vi "Swerve Controller.vi"(8 "error in":errorcluster) -> ()   [LabVIEW 2023]
doc: "This VI executes continuously carrying out the current operation and responding to updates or new operations. It will often contain the timing or control code that is difficult to place directly in TeleOp. This VI generally opens all sensors and motors and isolates the rest of the robot code from knowing how the operations are carried out."
uses:
  <vilib>/Rock Robotics/WPI/Framework/Completion Status.ctl
  Swerve Setpoints2.ctl
  Swerve Operations.ctl
  Framework/Robot Global Data.vi
  <vilib>/addons/control/pid/pid.llb/PID (DBL).vi
  <vilib>/addons/control/pid/NI_PID_pid.lvlib
  <vilib>/Rock Robotics/Network Tables/NT Write Boolean.vi
panel:
  out "error out":errorcluster
  out "x-y":u32
  in  "Tape":T1={"proportional gain (Kc)"=1.0, "integral time (Ti, min)"=0.01, "derivative time (Td, min)"=0.0} {"derivative time (Td, min)" format="%.3f"; "integral time (Ti, min)" format="%.3f"; "proportional gain (Kc)" format="%.3f"}
  in  "AprilTag":T1={"proportional gain (Kc)"=1.0, "integral time (Ti, min)"=0.01, "derivative time (Td, min)"=0.0} {"derivative time (Td, min)" format="%.3f"; "integral time (Ti, min)" format="%.3f"; "proportional gain (Kc)" format="%.3f"}
  in  "Look At Cube":T1={"proportional gain (Kc)"=0.001, "integral time (Ti, min)"=0.0, "derivative time (Td, min)"=0.0}
  in  "Look At Cone":T1={"proportional gain (Kc)"=0.004, "integral time (Ti, min)"=0.0, "derivative time (Td, min)"=0.01}
  in  "Balance":T1={"proportional gain (Kc)"=0.011, "integral time (Ti, min)"=0.0, "derivative time (Td, min)"=0.0} {"derivative time (Td, min)" format="%.3f"; "integral time (Ti, min)" format="%.3f"; "proportional gain (Kc)" format="%.3f"}
  in  "Drive to Angle(Distance)":T1={"proportional gain (Kc)"=0.9, "integral time (Ti, min)"=0.0, "derivative time (Td, min)"=0.0} {"derivative time (Td, min)" format="%.3f"; "integral time (Ti, min)" format="%.3f"; "proportional gain (Kc)" format="%.3f"}
  in  "Drive to Angle(Distance)":T1={"proportional gain (Kc)"=0.022, "integral time (Ti, min)"=0.0, "derivative time (Td, min)"=0.0} {"derivative time (Td, min)" format="%.3f"; "integral time (Ti, min)" format="%.3f"; "proportional gain (Kc)" format="%.3f"}
  out "Gyro":dbl
  in  "Drive to angle(Time)":T1={"proportional gain (Kc)"=0.019999999999999574, "integral time (Ti, min)"=0.0, "derivative time (Td, min)"=0.0} {"derivative time (Td, min)" format="%.3f"; "integral time (Ti, min)" format="%.3f"; "proportional gain (Kc)" format="%.3f"}
  in  "Turn to Angle":T1={"proportional gain (Kc)"=0.019999999999999574, "integral time (Ti, min)"=0.0, "derivative time (Td, min)"=0.0} {"derivative time (Td, min)" format="%.3f"; "integral time (Ti, min)" format="%.3f"; "proportional gain (Kc)" format="%.3f"}
  in  "Interactive Values":T2
  out "Current\nCmd":string="Started at  16:27:40.452\nDefault: Reserve,  S 0.0, D 0.000000"
  in  "Buttons":cluster{"Execute Cmd":bool, "Abort Cmd":bool}
  out "Command Timing":cluster{"Start Time (ms)":u32, "Iterations":i32}={"Start Time (ms)"=1585114, "Iterations"=-1}
  out "Status":T4=enum."Aborted"
  # "Tip: It may be helpful to observe inputs and sensor values.\nYou may also want to display tuning or debugging controls."
  # "Interactive Command: You may fill in the settings for a command\nand schedule it with the Execute button. You can observe and abort\nany command while fine tuning the code for the controller."
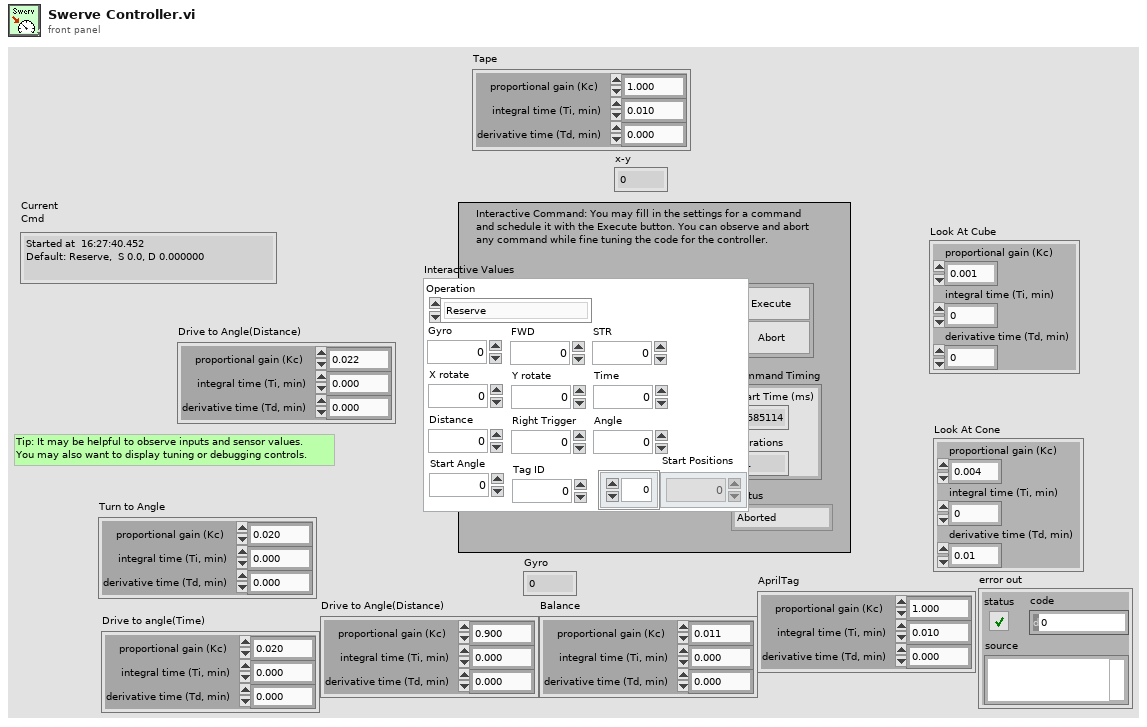
[diagram p1: front panel]
types:
  T1 = cluster{"proportional gain (Kc)":dbl, "integral time (Ti, min)":dbl, "derivative time (Td, min)":dbl}
  T2 = typedef "Swerve Setpoints2.ctl" = cluster{"Operation":T3, "Gyro":dbl, "FWD":dbl, "STR":dbl, "X rotate":dbl, "Y rotate":dbl, "Time":dbl, "Distance":dbl, "Right Trigger":dbl, "Angle":dbl, "Start Angle":dbl, "Tag ID":dbl, "Start Positions":dbl[]}
  T3 = typedef "Swerve Operations.ctl" = enum16{"Reserve", "Read Current", "Immediate", "Stop", "Balance", "Direct  Joystick Drive", "Joystick Drive", "Drive for Distance", "Drive for Time", "Turn to Angle", "Drive to Angle(Time)", "Drive to Angle(Distance)", "Look At Cone", "Look At Cube", "Move To Tape", "Move To Tag"}
  T4 = typedef "Completion Status.ctl" = enum16{"Successful", "Aborted", "Incomplete"}
  T5 = typedef "Command Status Info.ctl" = cluster{"Name":string, "Status":T4, "notifier out":T6}
  T6 = typedef "Completion Notifier.ctl" = refnum<notifier>
  T7 = cluster{"Current Command":T2, "Command Timing":cluster{"Start Time (ms)":u32, "Iterations":i32}, "Command Arguments":cluster{"Command Info":T5, "Description":string, "Default Command":T2, "queue out":refnum<queue>, "Subsystem Name":string}}
  T8 = enum16{"AprilTag", "Reflective Tape", "Custom", "Cube", "Cone"}
  T9 = typedef "ADIS16470 Device Reference.ctl" = cluster{"DevStatus":errorcluster, "Hardware Config":T10, "Calibration Complete":refnum<notifier>, "Status Reference":refnum<data-value>, "Data Reference":refnum<data-value>, "Sychronous Process VI":T14, "Cmd FIFO":refnum<k33>, "Source":T15, "Data FIFO":refnum<k33>, "Calibration Time (ms)":u32, "Data Reference":refnum<data-value>}
  T10 = typedef "ADIS16470 Hardware Configuration.ctl" = cluster{"SPI Clock Rate (Hz)":dbl, "IMU SPI Mode (3)":T11, "IMU Reset Pin":T12, "IMU SPI Bus":T13, "IMU Data Ready Pin":T12, "Stall Config":cluster{"Pow2BytesPerRead":u8, "StallTicks":u16, "CsToSclkTicks":u8}}
  T11 = typedef "WPI_SPIMode.ctl" = enum16{"Mode 0 (Clk Idle Low,Sample on Leading)", "Mode 1 (Clk Idle Low,Sample on Trailing)", "Mode 2 (Clk Idle High,Sample on Leading)", "Mode 3 (Clk Idle High,Sample on Trailing)"}
  T12 = typedef "FPGA_DIOChannel.ctl" = enum8{"DIO 0", "DIO 1", "DIO 2", "DIO 3", "DIO 4", "DIO 5", "DIO 6", "DIO 7", "DIO 8", "DIO 9", "DIO MXP 0", "DIO MXP 1", "DIO MXP 2", "DIO MXP 3", "DIO MXP 4", "DIO MXP 5", "DIO MXP 6", "DIO MXP 7", "DIO MXP 8", "DIO MXP 9", "DIO MXP 10", "DIO MXP 11", "DIO MXP 12", "DIO MXP 13", "DIO MXP 14", "DIO MXP 15", "SPI Port CS1", "SPI Port CS2", "SPI Port CS3", "SPI Port MISO", "SPI Port MOSI", "Invalid"}
  T13 = typedef "spi_bus.ctl" = enum16{"SPI On-Board, CS0", "SPI On-Board, CS1", "SPI On-Board, CS2", "SPI On-Board, CS3", "SPI MXP", "Invalid"}
  T14 = typedef "ADIS16470 Process.ctl" = refnum<vi>
  T15 = typedef "FPGA_CounterEncoderSourceConvertionLVSourceType.ctl" = cluster{"DevStatus":errorcluster, "AnalogTriggerMode?":bool, "DigitalMode":cluster{"DIO Channel":T16}, "AnalogTriggerMode":cluster{"AnalogTriggerIndex":T17, "OutputType":T18}}
  T16 = typedef "FPGA_DIODigitalSourceChannel.ctl" = enum8{"DIO 0", "DIO 1", "DIO 2", "DIO 3", "DIO 4", "DIO 5", "DIO 6", "DIO 7", "DIO 8", "DIO 9", "DIO MXP 0", "DIO MXP 1", "DIO MXP 2", "DIO MXP 3", "DIO MXP 4", "DIO MXP 5", "DIO MXP 6", "DIO MXP 7", "DIO MXP 8", "DIO MXP 9", "DIO MXP 10", "DIO MXP 11", "DIO MXP 12", "DIO MXP 13", "DIO MXP 14", "DIO MXP 15", "SPI Port CS1", "SPI Port CS2", "SPI Port CS3", "SPI Port MISO", "SPI Port MOSI", "Disabled"}
  T17 = typedef "FPGA_AnalogTriggerIndex.ctl" = enum8{"Trig 0", "Trig 1", "Trig 2", "Trig 3", "Trig 4", "Trig 5", "Trig 6", "Trig 7", "Invalid"}
  T18 = typedef "FPGA_AnalogTriggerOutType.ctl" = enum16{"InWindow", "TriggerState", "Rising", "Falling"}
  T19 = typedef "ADIS16470 Data.ctl" = cluster{"XAngle":dbl, "YAngle":dbl, "ZAngle":dbl}
  T20 = typedef "WPI_MotorControlDeviceRef.ctl" = cluster{"DeviceStatus":errorcluster, "Type":T21, "PWM":cluster{"PWM Channel":T22, "DeadBand":T23}, "CAN":cluster{"Device Number":u8, "SetOutput VI Ref":variant, "GetOutput VI Ref":variant, "Enable VI Ref":variant, "Disable VI Ref":variant, "Data":variant}, "Invert":bool, "DIO PWM":cluster{"PWM \"Enable\" Channel":T22, "DIOChannel":T12, "PWM Rate":dbl}}
  T21 = typedef "WPI_MotorControlType.ctl" = enum16{"PWM", "CAN", "DIO PWM"}
  T22 = typedef "FPGA_DIOPWMChannel.ctl" = enum8{"PWM 0", "PWM 1", "PWM 2", "PWM 3", "PWM 4", "PWM 5", "PWM 6", "PWM 7", "PWM 8", "PWM 9", "PWM MXP 0", "PWM MXP 1", "PWM MXP 2", "PWM MXP 3", "PWM MXP 4", "PWM MXP 5", "PWM MXP 6", "PWM MXP 7", "PWM MXP 8", "PWM MXP 9", "Invalid"}
  T23 = typedef "WPI_PWMDeadband.ctl" = cluster{"Name":string, "maxPositivePwm":i32, "minPositivePwm":i32, "centerPwm":i32, "maxNegativePwm":i32, "minNegativePwm":i32, "angularRange":u16}
  T24 = cluster{"tag ID":i32, "Center":cluster{"X":dbl, "Y":dbl}, "homography matrix":dbl[], "decision margin":dbl, "Hamming Dist":i32, "corner points":cluster{"X":dbl, "Y":dbl}[], "Tag Family":string}[]
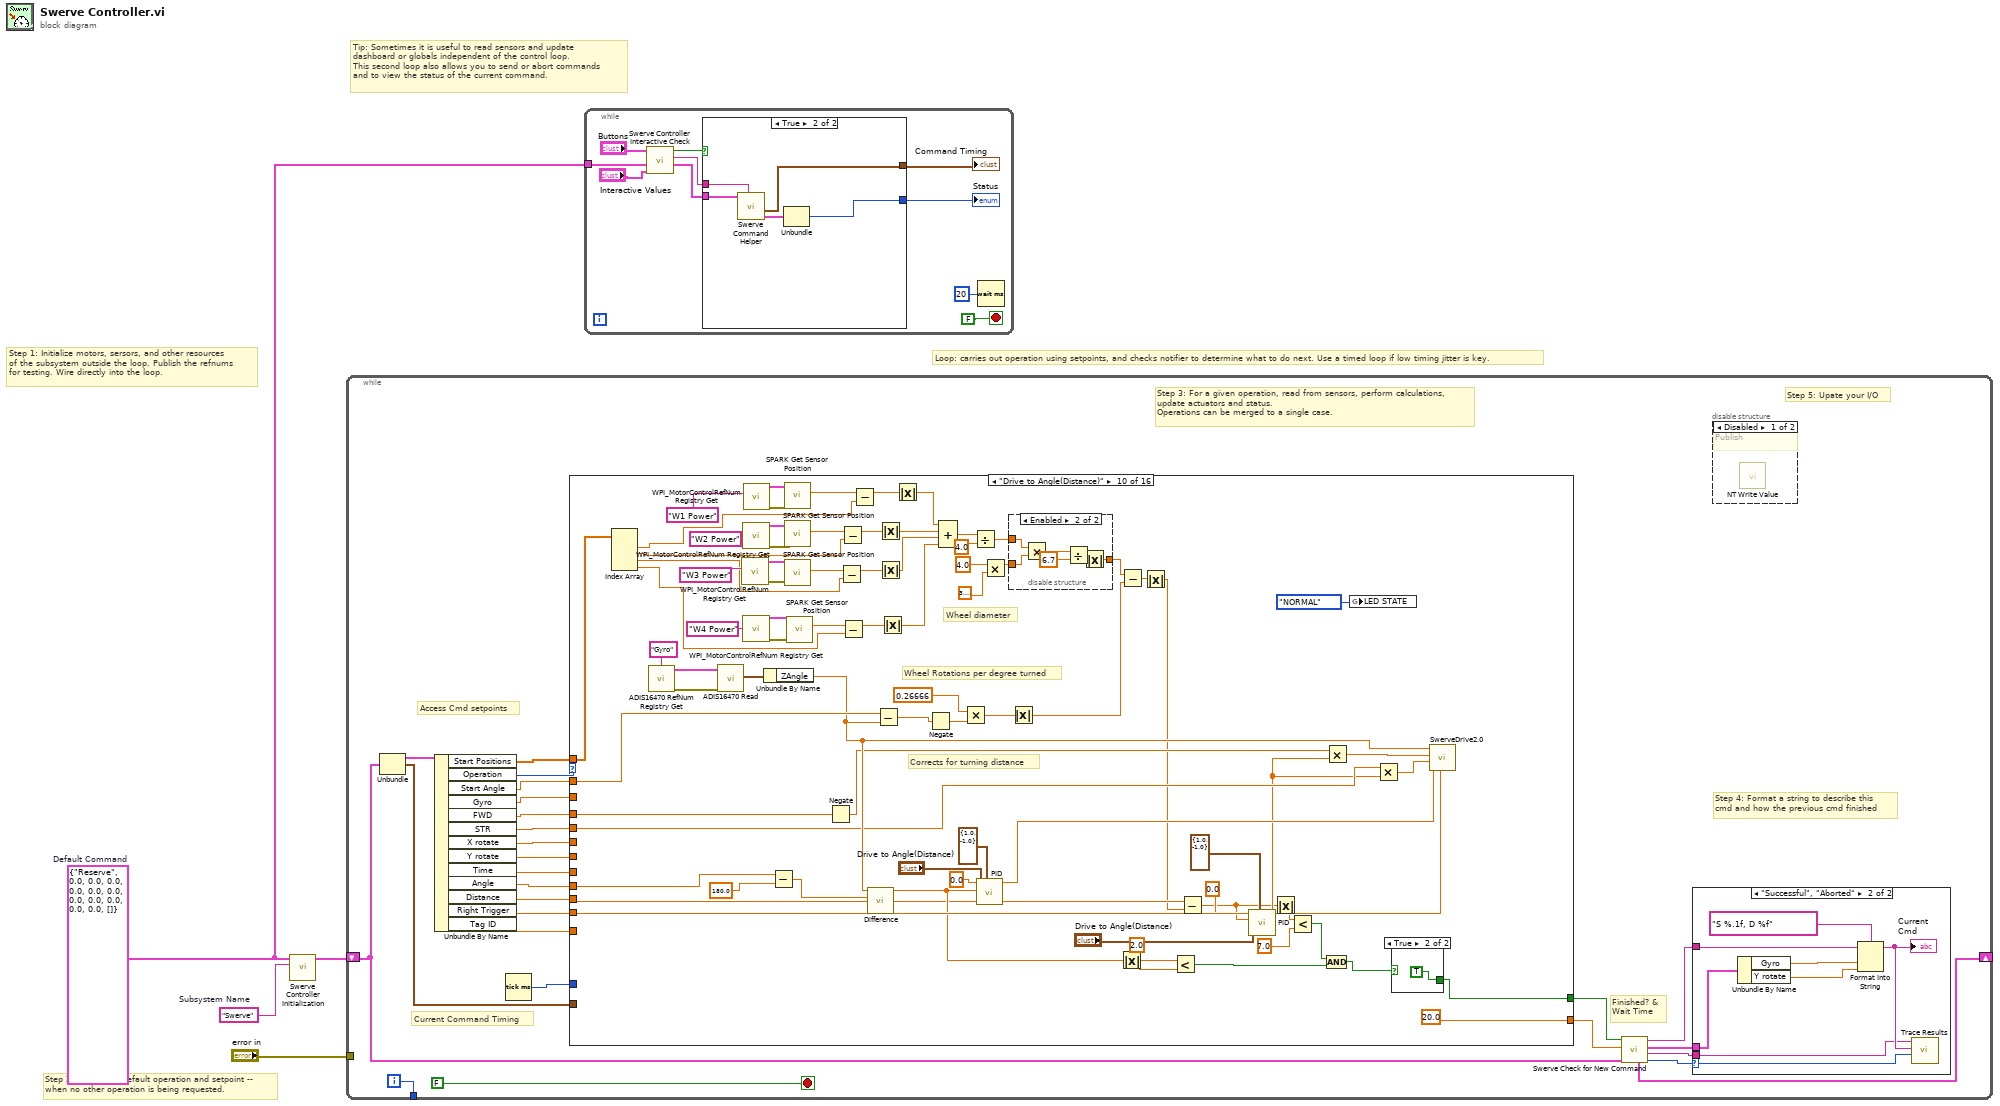
[diagram p0: block diagram]
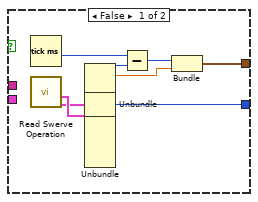
[diagram p2: hidden frame]
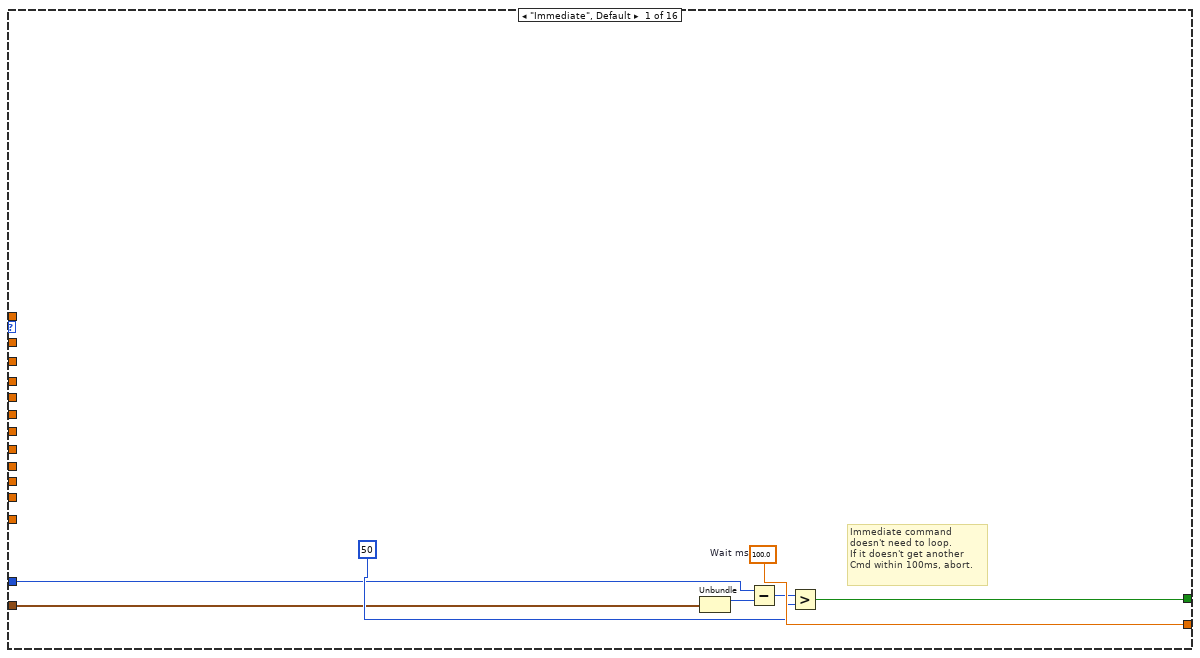
[diagram p3: hidden frame]
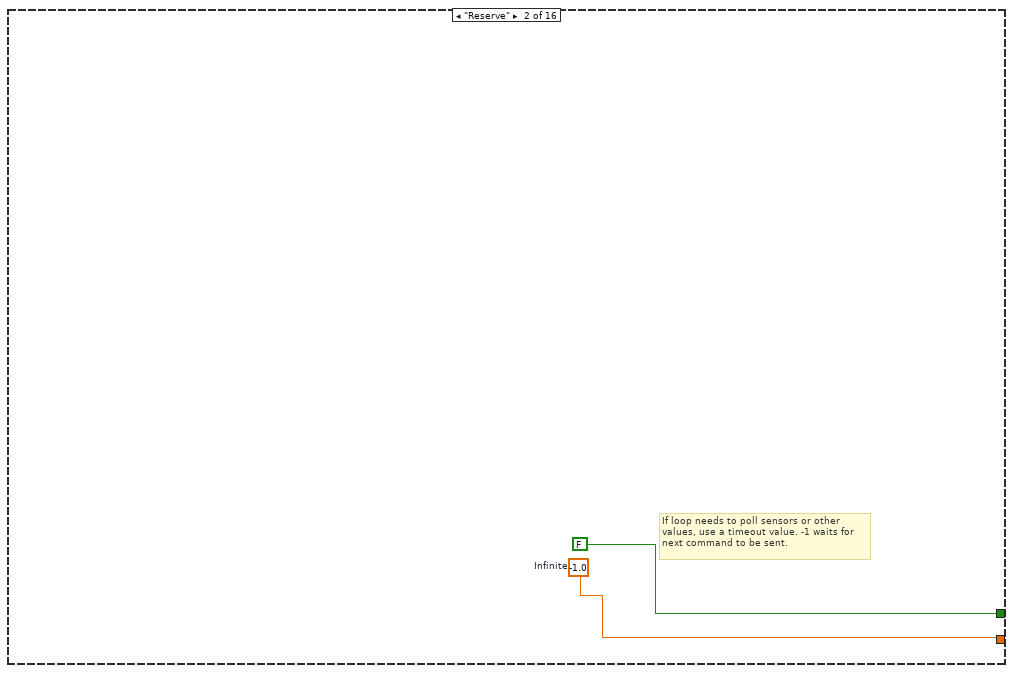
[diagram p4: hidden frame]
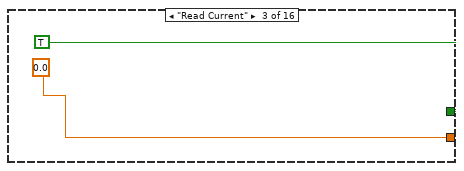
[diagram p5: hidden frame]
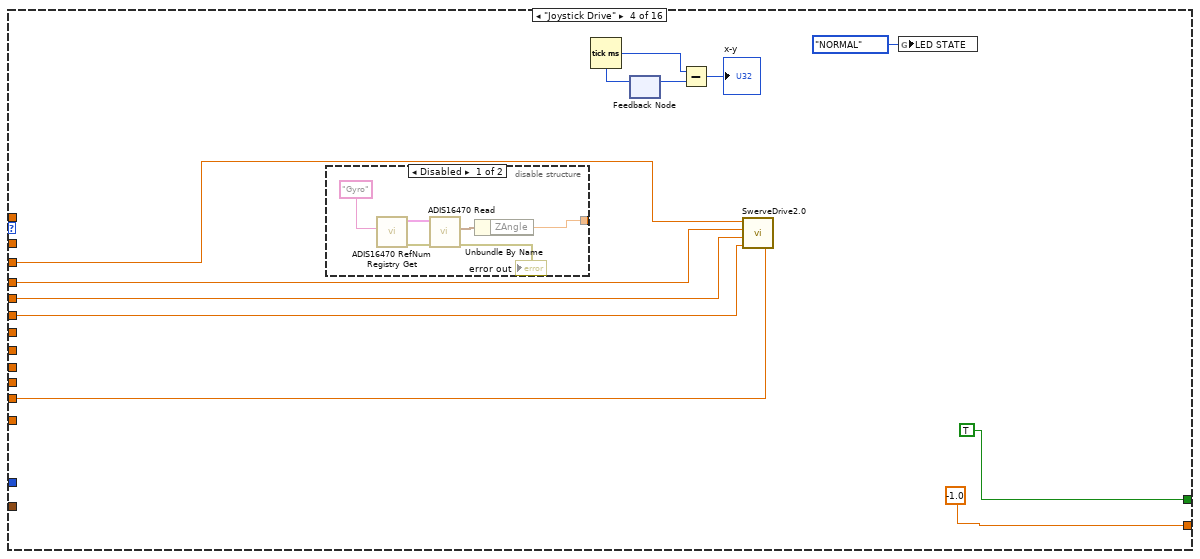
[diagram p6: hidden frame]
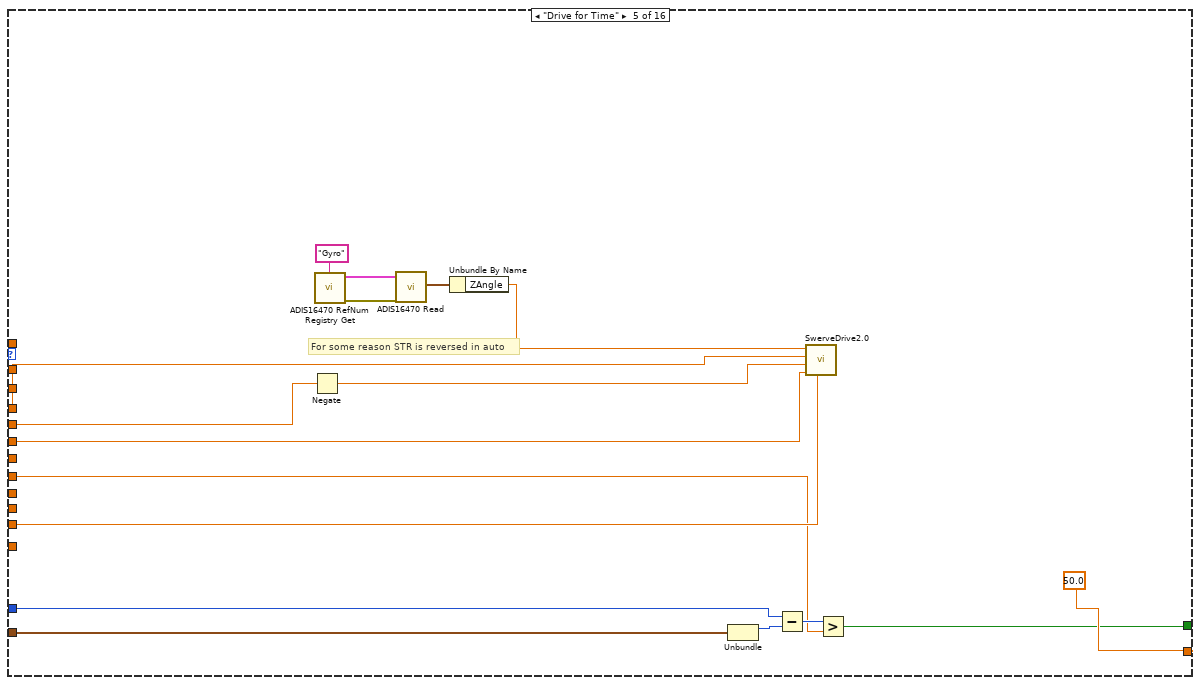
[diagram p8: hidden frame]
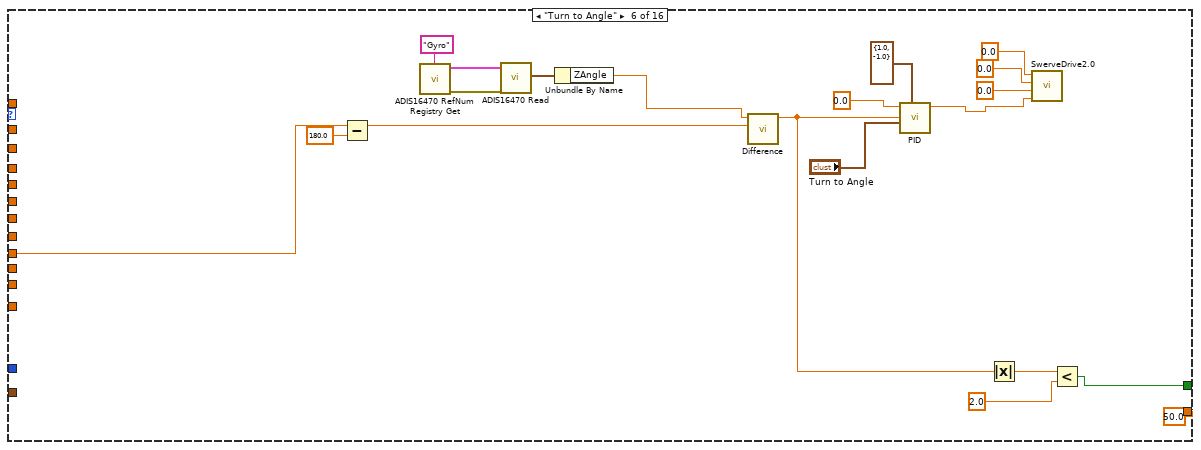
[diagram p9: hidden frame]
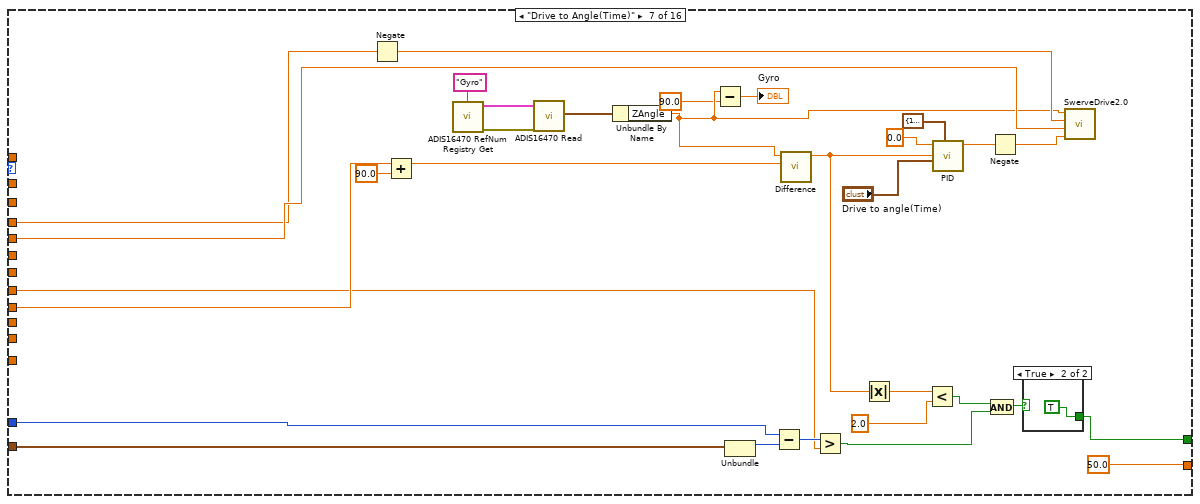
[diagram p10: hidden frame]
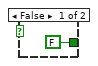
[diagram p11: hidden frame]
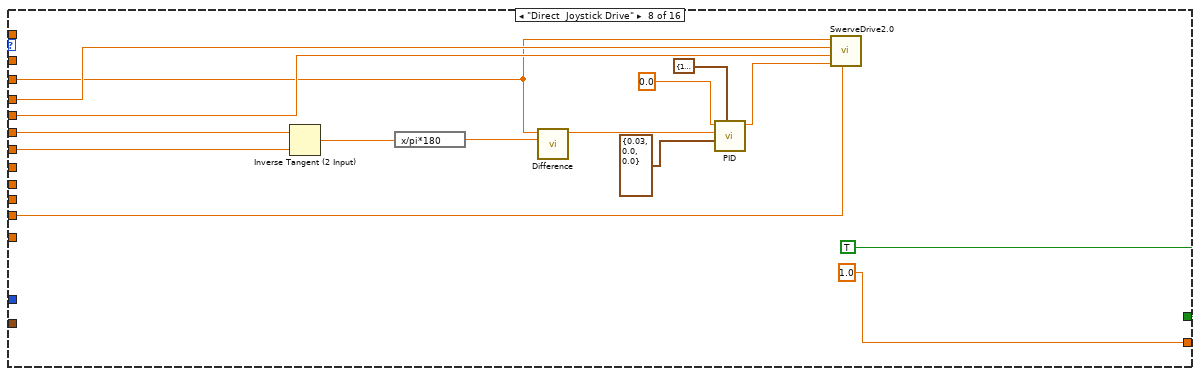
[diagram p12: hidden frame]
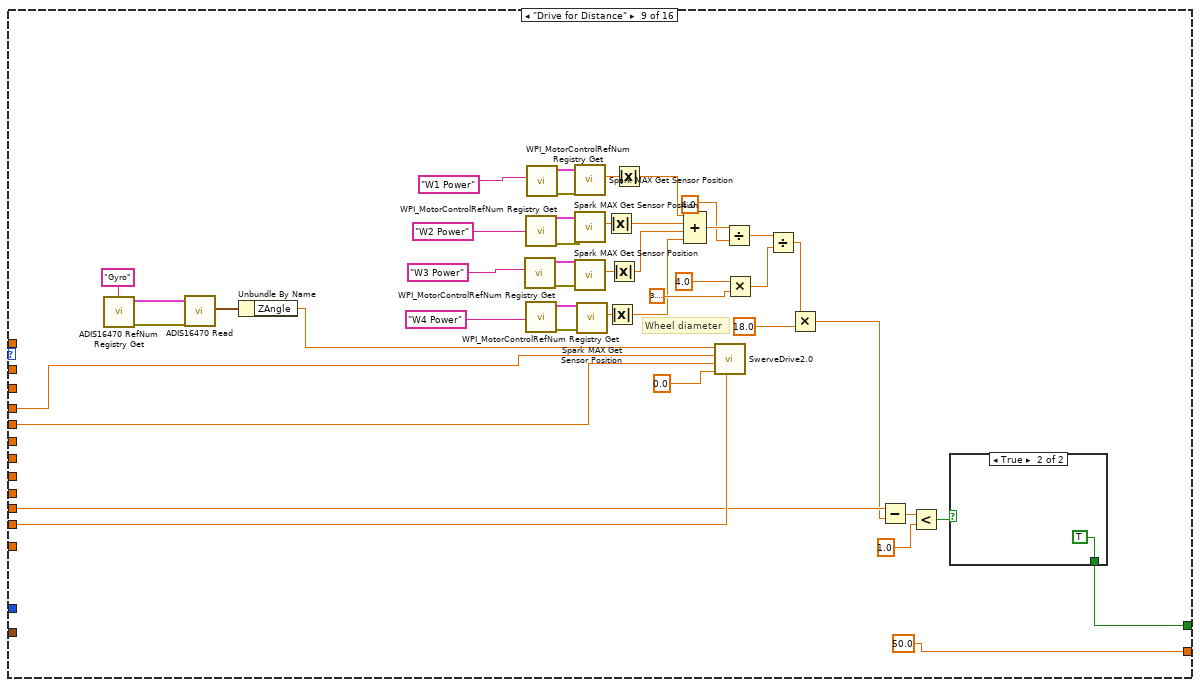
[diagram p13: hidden frame]
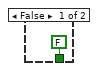
[diagram p14: hidden frame]
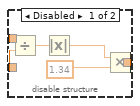
[diagram p15: hidden frame]
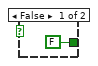
[diagram p16: hidden frame]
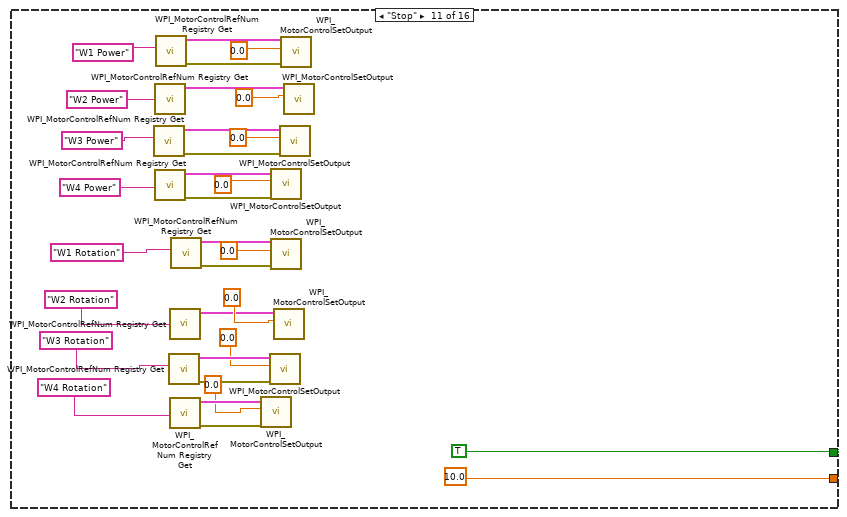
[diagram p17: hidden frame]
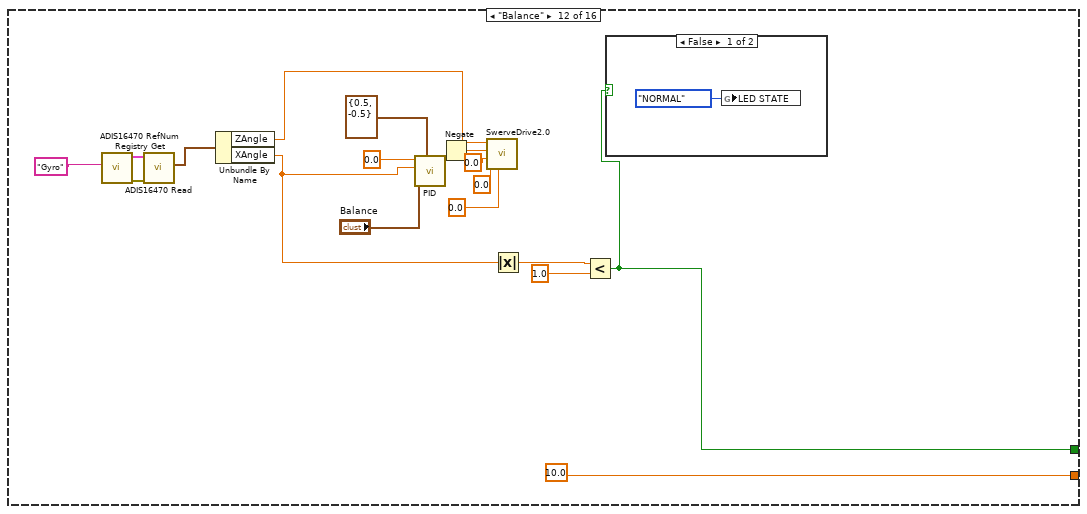
[diagram p18: hidden frame]
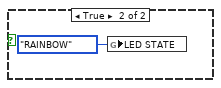
[diagram p19: hidden frame]
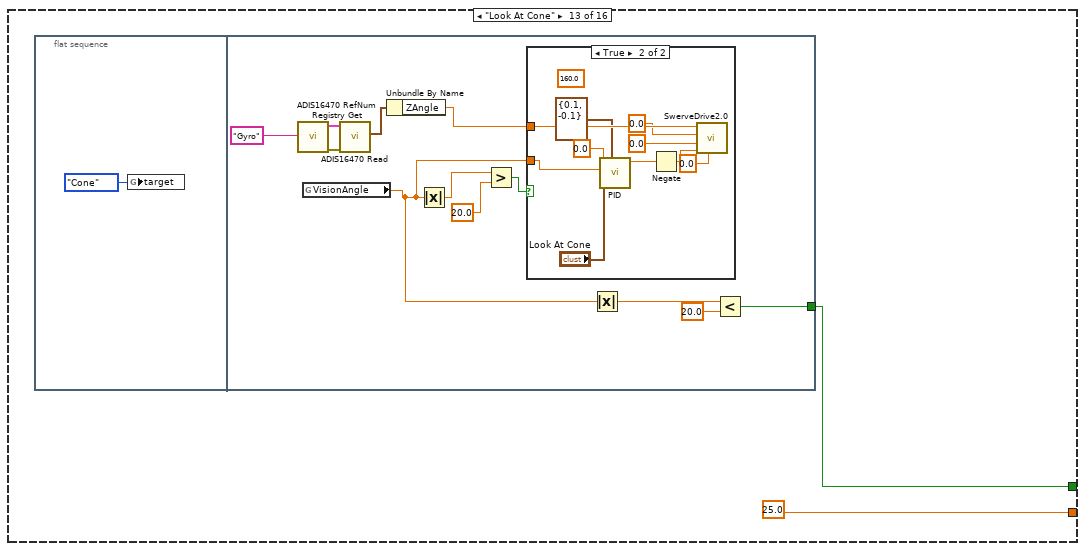
[diagram p20: hidden frame]
diagram:
  w1 = T2 {"Operation"=enum."Reserve", "Gyro"=0.0, "FWD"=0.0, "STR"=0.0, "X rotate"=0.0, "Y rotate"=0.0, "Time"=0.0, "Distance"=0.0, "Right Trigger"=0.0, "Angle"=0.0, "Start Angle"=0.0, "Tag ID"=0.0, "Start Positions"=[]}  # Default Command
  w2 = "Swerve"  # Subsystem Name
  # "Tip: Sometimes it is useful to read sensors and update\ndashboard or globals independent of the control loop.\nThis second loop also allows you to send or abort commands\nand to view the status of the current command."
  # "Step 2: Define the default operation and setpoint --\nwhen no other operation is being requested."
  # "Step 1: Initialize motors, sersors, and other resources\nof the subsystem outside the loop. Publish the refnums\nfor testing. Wire directly into the loop."
  # "Loop: carries out operation using setpoints, and checks notifier to determine what to do next. Use a timed loop if low timing jitter is key."
  n1 = call "Swerve Controller Initialization.vi"("Subsystem Name"=w2, "Default Command"=w1) -> ("Current Command"=w3:T7)  [unwired: 9 in]
  n2 = while {
    shift-right: [w24] -> _
    shift-left: w3 -> [w18]
    tunnel: [w29] -> _
    tunnel: "error in" -> [_]
    i -> [w29]
    stop <- FALSE stop-if-true
    # "Step 5: Upate your I/O"
    # "Step 4: Format a string to describe this\ncmd and how the previous cmd finished"
    # "Current Command Timing"
    # "Access Cmd setpoints"
    # "Finished? &\nWait Time"
    # "Step 3: For a given operation, read from sensors, perform calculations,\nupdate actuators and status.\nOperations can be merged to a single case."
    n3 = Unbundle(w18) -> ("Current Command"=w28:T2, "Command Timing"=w25:cluster{"Start Time (ms)":u32, "Iterations":i32})  [unwired: 1 out]
    n4 = Unbundle By Name(w28) -> ("Start Positions"=w5:dbl[], "Operation"=w27:T3, "Start Angle"=w8:dbl, "Gyro"=w17:dbl, "FWD"=w16:dbl, "STR"=w15:dbl, "X rotate"=w14:dbl, "Y rotate"=w9:dbl, "Time"=w10:dbl, "Angle"=w13:dbl, "Distance"=w12:dbl, "Right Trigger"=w11:dbl, "Tag ID"=w7:dbl)
    n5 = Tick Count (ms)() -> (millisecond timer value=w26:u32)
    n6 = case shown="\"Drive to Angle(Distance)\"" w27 {
      tunnel: [w37 w39 0.0 ("Time") -1.0 ("Infinite") 50.0 ("Time") 50.0 ("Time") 50.0 ("Time") 1.0 ("Time") 50.0 ("Time") 20.0 ("Time") 10.0 ("Time") 10.0 ("Time") 25.0 ("Time") 25.0 ("Time") 10.0 ("Time") 10.0 ("Time")] -> w23
      tunnel: w25 -> [w33 _ _ _ w69 _ w124 _ _ _ _ _ _ _ _ _]
      tunnel: w26 -> [w32 _ _ _ w70 _ w123 _ _ _ _ _ _ _ _ _]
      tunnel: w17 -> [_ _ _ w42 _ _ _ w130 _ _ _ _ _ _ _ _]
      tunnel: w16 -> [_ _ _ w52 w73 _ w103 w141 w145 w265 _ _ _ _ _ _]
      tunnel: w15 -> [_ _ _ w49 w74 _ w104 w142 w167 w205 _ _ _ _ _ _]
      tunnel: w14 -> [_ _ _ w48 w66 _ _ w136 _ _ _ _ _ _ _ _]
      tunnel: w13 -> [_ _ _ _ _ w80 w102 _ _ w264 _ _ _ _ _ _]
      tunnel: w12 -> [_ _ _ _ _ _ _ _ w165 w221 _ _ _ _ _ _]
      tunnel: w11 -> [_ _ _ w51 w75 _ _ w143 w187 w266 _ _ _ _ _ _]
      tunnel: w10 -> [_ _ _ _ w67 _ w101 _ _ _ _ _ _ _ _ _]
      tunnel: w9 -> [_ _ _ _ _ _ _ w135 _ _ _ _ _ _ _ _]
      tunnel: w8 -> [_ _ _ _ _ _ _ _ _ w217 _ _ _ _ _ _]
      tunnel: w7 -> [_ _ _ _ _ _ _ _ _ _ _ _ _ _ w389 _]
      tunnel: [w31 FALSE ("ignore previous (F)") TRUE ("ignore previous (F)") TRUE ("ignore previous (F)") w59 w76 w96 TRUE ("ignore previous (F)") w144 w203 TRUE ("ignore previous (F)") w315 w335 w360 w388 w424] -> w6
      tunnel: w5 -> [_ _ _ _ _ _ _ _ _ w196 _ _ _ _ _ _]
      frame "Immediate", Default {
        w37 = 100.0  # Wait ms
        # "Immediate command\ndoesn't need to loop.\nIf it doesn't get another\nCmd within 100ms, abort."
        n7 = Unbundle(w33) -> ("Start Time (ms)"=w36:u32)  [unwired: 1 out]
        n8 = Subtract(x=w32, y=w36) -> (x-y=w35:u32)
        n9 = Greater?(x=w35, y=u8 50 ("Left Motor")) -> (0:w31:bool)
      }
      frame "Reserve" {
        w39 = -1.0  # Infinite
        # "If loop needs to poll sensors or other\nvalues, use a timeout value. -1 waits for\nnext command to be sent."
      }
      frame "Read Current" {
      }
      frame "Joystick Drive" {
        n10 = disable-structure shown="Disabled" {
          disable-tunnel: [w54 _] -> _
          frame Disabled {
            n11 = call <vilib>:"ADIS16470 RefNum Registry Get.vi"("refnum name"="Gyro") -> ("error out"=w58:errorcluster, "ADIS16470DevRef out"=w57:T9)  [unwired: 9 in]
            n12 = call <vilib>:"ADIS16470 Read.vi"("error in (no error)"=w58, "ADIS16470DevRef"=w57) -> ("error out"=→"error out":errorcluster, "ADIS16470 Value"=w55:T19)  [unwired: 6 in, 2 out]
            n13 = Unbundle By Name(w55) -> ("ZAngle"=w54:dbl)
          }
          frame Enabled {
          }
        }
        n14 = Tick Count (ms)() -> (millisecond timer value=w46:u32)
        n15 = feedback-in #1(w46) -> ()
        n16 = feedback #1() -> (w45:u32)  [unwired: 1 in]
        n17 = Subtract(x=w46, y=w45) -> (x-y=→"x-y":u32)
        n18 = call "SwerveDrive2.0.vi"("Right Trigger"=w51, "RCW"=w48, "STR"=w49, "FWD"=w52, "Gyro"=w42) -> ()  [unwired: 7 in]
        n19 = global write "Robot Global Data.vi" "LED STATE"(enum16{"NORMAL", "RAINBOW"}."NORMAL" ("LED STATE")) -> ()
      }
      frame "Drive for Time" {
        # "For some reason STR is reversed in auto"
        n20 = Negate(x=w74) -> (-x=w60:dbl)
        n21 = call <vilib>:"ADIS16470 RefNum Registry Get.vi"("refnum name"="Gyro") -> ("error out"=w65:errorcluster, "ADIS16470DevRef out"=w64:T9)  [unwired: 9 in]
        n22 = call <vilib>:"ADIS16470 Read.vi"("error in (no error)"=w65, "ADIS16470DevRef"=w64) -> ("ADIS16470 Value"=w63:T19)  [unwired: 6 in, 3 out]
        n23 = Unbundle By Name(w63) -> ("ZAngle"=w61:dbl)
        n24 = Unbundle(w69) -> ("Start Time (ms)"=w72:u32)  [unwired: 1 out]
        n25 = Subtract(x=w70, y=w72) -> (x-y=w71:u32)
        n26 = call "SwerveDrive2.0.vi"("Right Trigger"=w75, "RCW"=w66, "STR"=w60, "FWD"=w73, "Gyro"=w61) -> ()  [unwired: 7 in]
        n27 = Greater?(x=w71, y=w67) -> (0:w59:bool)
      }
      frame "Turn to Angle" {
        n28 = Subtract(x=w80, y=180.0) -> (x-y=w79:dbl)
        n29 = call <vilib>:"ADIS16470 RefNum Registry Get.vi"("refnum name"="Gyro") -> ("error out"=w90:errorcluster, "ADIS16470DevRef out"=w89:T9)  [unwired: 9 in]
        n30 = call <vilib>:"ADIS16470 Read.vi"("error in (no error)"=w90, "ADIS16470DevRef"=w89) -> ("ADIS16470 Value"=w88:T19)  [unwired: 6 in, 3 out]
        n31 = Unbundle By Name(w88) -> ("ZAngle"=w86:dbl)
        n32 = call "Difference.vi"("Angle"=w79, "Gyro"=w86) -> ("Difference"=w84:dbl)  [unwired: 9 in]
        n33 = call-poly <vilib>:"PID.vi"("output range"=cluster{"output high":dbl, "output low":dbl} {"output high"=1.0, "output low"=-1.0}, "PID gains"="Turn to Angle", "process variable"=w84, "setpoint"=0.0) -> ("output"=w77:dbl)  [unwired: 6 in, 1 out]
        n34 = Absolute Value(x=w84) -> (abs(x)=w82:dbl)
        n35 = call "SwerveDrive2.0.vi"("RCW"=w77, "STR"=0.0, "FWD"=0.0, "Gyro"=0.0) -> ()  [unwired: 8 in]
        n36 = Less?(x=w82, y=2.0) -> (x < y?=w76:bool)
      }
      frame "Drive to Angle(Time)" {
        n37 = Negate(x=w103) -> (-x=w100:dbl)
        n38 = Add(x=w102, y=90.0) -> (x+y=w111:dbl)
        n39 = call <vilib>:"ADIS16470 RefNum Registry Get.vi"("refnum name"="Gyro") -> ("error out"=w116:errorcluster, "ADIS16470DevRef out"=w115:T9)  [unwired: 9 in]
        n40 = call <vilib>:"ADIS16470 Read.vi"("error in (no error)"=w116, "ADIS16470DevRef"=w115) -> ("ADIS16470 Value"=w114:T19)  [unwired: 6 in, 3 out]
        n41 = Unbundle By Name(w114) -> ("ZAngle"=w99:dbl)
        n42 = Subtract(x=w99, y=90.0) -> (x-y=→"Gyro":dbl)
        n43 = Unbundle(w124) -> ("Start Time (ms)"=w126:u32)  [unwired: 1 out]
        n44 = Subtract(x=w123, y=w126) -> (x-y=w125:u32)
        n45 = call "Difference.vi"("Angle"=w111, "Gyro"=w99) -> ("Difference"=w108:dbl)  [unwired: 9 in]
        n46 = Greater?(x=w125, y=w101) -> (0:w121:bool)
        n47 = Absolute Value(x=w108) -> (abs(x)=w106:dbl)
        n48 = Less?(x=w106, y=2.0) -> (x < y?=w105:bool)
        n49 = call-poly <vilib>:"PID.vi"("output range"=cluster{"output high":dbl, "output low":dbl} {"output high"=1.0, "output low"=-1.0}, "PID gains"="Drive to angle(Time)", "process variable"=w108, "setpoint"=0.0) -> ("output"=w117:dbl)  [unwired: 6 in, 1 out]
        n50 = And(x=w105, y=w121) -> (x .and. y?=w122:bool)
        n51 = Negate(x=w117) -> (-x=w109:dbl)
        n52 = case shown="True" w122 {
          tunnel: [FALSE ("ignore previous (F)") TRUE ("ignore previous (F)")] -> w96
          frame False {
          }
          frame True {
          }
        }
        n53 = call "SwerveDrive2.0.vi"("RCW"=w109, "STR"=w104, "FWD"=w100, "Gyro"=w99) -> ()  [unwired: 8 in]
      }
      frame "Direct  Joystick Drive" {
        n54 = Inverse Tangent (2 Input)(1:w135, 2:w136) -> (0:w133:dbl)
        n55 = expression code="x/pi*180"(w133) -> (w131:dbl)
        n56 = call "Difference.vi"("Angle"=w131, "Gyro"=w130) -> ("Difference"=w132:dbl)  [unwired: 9 in]
        n57 = call-poly <vilib>:"PID.vi"("output range"=cluster{"output high":dbl, "output low":dbl} {"output high"=1.0, "output low"=-1.0}, "PID gains"=T1 {"proportional gain (Kc)"=0.03, "integral time (Ti, min)"=0.0, "derivative time (Td, min)"=0.0}, "process variable"=w132, "setpoint"=0.0) -> ("output"=w140:dbl)  [unwired: 6 in, 1 out]
        n58 = call "SwerveDrive2.0.vi"("Right Trigger"=w143, "RCW"=w140, "STR"=w142, "FWD"=w141, "Gyro"=w130) -> ()  [unwired: 7 in]
      }
      frame "Drive for Distance" {
        # "Wheel diameter"
        n59 = call <vilib>:"ADIS16470 RefNum Registry Get.vi"("refnum name"="Gyro") -> ("error out"=w162:errorcluster, "ADIS16470DevRef out"=w161:T9)  [unwired: 9 in]
        n60 = call <vilib>:"ADIS16470 Read.vi"("error in (no error)"=w162, "ADIS16470DevRef"=w161) -> ("ADIS16470 Value"=w160:T19)  [unwired: 6 in, 3 out]
        n61 = Unbundle By Name(w160) -> ("ZAngle"=w158:dbl)
        n62 = call <vilib>:"WPI_MotorControlRefNum Registry Get.vi"("refnum name"="W3 Power") -> ("error out"=w181:errorcluster, "MotorControlDevRef"=w180:T20)  [unwired: 9 in]
        n63 = call <vilib>:"WPI_MotorControlRefNum Registry Get.vi"("refnum name"="W2 Power") -> ("error out"=w183:errorcluster, "MotorControlDevRef"=w182:T20)  [unwired: 9 in]
        n64 = call <vilib>:"WPI_MotorControlRefNum Registry Get.vi"("refnum name"="W4 Power") -> ("error out"=w179:errorcluster, "MotorControlDevRef"=w178:T20)  [unwired: 9 in]
        n65 = call <vilib>:"WPI_MotorControlRefNum Registry Get.vi"("refnum name"="W1 Power") -> ("error out"=w185:errorcluster, "MotorControlDevRef"=w184:T20)  [unwired: 9 in]
        n66 = call <vilib>:"Spark MAX Get Sensor Position.vi"("error in (no error)"=w185, "MotorControlDevRef in"=w184) -> ("Sensor Position"=w170:dbl)  [unwired: 6 in, 3 out]
        n67 = call <vilib>:"Spark MAX Get Sensor Position.vi"("error in (no error)"=w183, "MotorControlDevRef in"=w182) -> ("Sensor Position"=w171:dbl)  [unwired: 6 in, 3 out]
        n68 = call <vilib>:"Spark MAX Get Sensor Position.vi"("error in (no error)"=w181, "MotorControlDevRef in"=w180) -> ("Sensor Position"=w172:dbl)  [unwired: 6 in, 3 out]
        n69 = call <vilib>:"Spark MAX Get Sensor Position.vi"("error in (no error)"=w179, "MotorControlDevRef in"=w178) -> ("Sensor Position"=w173:dbl)  [unwired: 6 in, 3 out]
        n70 = Absolute Value(x=w171) -> (abs(x)=w153:dbl)
        n71 = Absolute Value(x=w173) -> (abs(x)=w151:dbl)
        n72 = Absolute Value(x=w172) -> (abs(x)=w152:dbl)
        n73 = Absolute Value(x=w170) -> (abs(x)=w154:dbl)
        n74 = Compound Arithmetic op=ADD(w154, w153, w152, w151) -> (w169:dbl)
        n75 = call "SwerveDrive2.0.vi"("Right Trigger"=w187, "RCW"=0.0, "STR"=w167, "FWD"=w145, "Gyro"=w158) -> ()  [unwired: 7 in]
        n76 = Divide(x=w169, y=4.0) -> (x/y=w164:dbl)
        n77 = Multiply(x=4.0 ("y"), y=3.141592653589793) -> (x*y=w155:dbl)
        n78 = Divide(x=w164, y=w155) -> (x/y=w163:dbl)
        n79 = Multiply(x=w163, y=18.0) -> (x*y=w150:dbl)
        n80 = Subtract(x=w165, y=w150) -> (x-y=w147:dbl)
        n81 = Less?(x=w147, y=1.0) -> (x < y?=w148:bool)
        n82 = case shown="True" w148 {
          tunnel: [FALSE ("ignore previous (F)") TRUE ("ignore previous (F)")] -> w144
          frame False {
          }
          frame True {
          }
        }
      }
      frame "Drive to Angle(Distance)" {
        # "Corrects for turning distance"
        # "Wheel Rotations per degree turned"
        # "Wheel diameter"
        n83 = Index Array(array=w196) -> (element #1=w195:dbl, element #2=w194:dbl, element #3=w193:dbl, element #4=w192:dbl)  [unwired: 4 in]
        n84 = call <vilib>:"ADIS16470 RefNum Registry Get.vi"("refnum name"="Gyro") -> ("error out"=w238:errorcluster, "ADIS16470DevRef out"=w237:T9)  [unwired: 9 in]
        n85 = call <vilib>:"ADIS16470 Read.vi"("error in (no error)"=w238, "ADIS16470DevRef"=w237) -> ("ADIS16470 Value"=w236:T19)  [unwired: 6 in, 3 out]
        n86 = call <vilib>:"WPI_MotorControlRefNum Registry Get.vi"("refnum name"="W3 Power") -> ("error out"=w258:errorcluster, "MotorControlDevRef"=w257:T20)  [unwired: 9 in]
        n87 = call <vilib>:"WPI_MotorControlRefNum Registry Get.vi"("refnum name"="W2 Power") -> ("error out"=w260:errorcluster, "MotorControlDevRef"=w259:T20)  [unwired: 9 in]
        n88 = call <vilib>:"WPI_MotorControlRefNum Registry Get.vi"("refnum name"="W4 Power") -> ("error out"=w256:errorcluster, "MotorControlDevRef"=w255:T20)  [unwired: 9 in]
        n89 = call <vilib>:"WPI_MotorControlRefNum Registry Get.vi"("refnum name"="W1 Power") -> ("error out"=w262:errorcluster, "MotorControlDevRef"=w261:T20)  [unwired: 9 in]
        n90 = Unbundle By Name(w236) -> ("ZAngle"=w216:dbl)
        n91 = Subtract(x=w264, y=180.0) -> (x-y=w228:dbl)
        n92 = call <vilib>:"SPARK Get Sensor Position.vi"("error in (no error)"=w262, "MotorControlDevRef in"=w261) -> ("Sensor Position"=w247:dbl)  [unwired: 6 in, 3 out]
        n93 = call <vilib>:"SPARK Get Sensor Position.vi"("error in (no error)"=w260, "MotorControlDevRef in"=w259) -> ("Sensor Position"=w248:dbl)  [unwired: 6 in, 3 out]
        n94 = call <vilib>:"SPARK Get Sensor Position.vi"("error in (no error)"=w258, "MotorControlDevRef in"=w257) -> ("Sensor Position"=w249:dbl)  [unwired: 6 in, 3 out]
        n95 = call <vilib>:"SPARK Get Sensor Position.vi"("error in (no error)"=w256, "MotorControlDevRef in"=w255) -> ("Sensor Position"=w250:dbl)  [unwired: 6 in, 3 out]
        n96 = Negate(x=w265) -> (-x=w208:dbl)
        n97 = Subtract(x=w249, y=w193) -> (x-y=w198:dbl)
        n98 = Subtract(x=w248, y=w194) -> (x-y=w199:dbl)
        n99 = Subtract(x=w250, y=w192) -> (x-y=w197:dbl)
        n100 = Subtract(x=w247, y=w195) -> (x-y=w200:dbl)
        n101 = call "Difference.vi"("Angle"=w228, "Gyro"=w216) -> ("Difference"=w229:dbl)  [unwired: 9 in]
        n102 = Subtract(x=w217, y=w216) -> (x-y=w218:dbl)
        n103 = Absolute Value(x=w199) -> (abs(x)=w225:dbl)
        n104 = Absolute Value(x=w198) -> (abs(x)=w224:dbl)
        n105 = Absolute Value(x=w197) -> (abs(x)=w223:dbl)
        n106 = Absolute Value(x=w200) -> (abs(x)=w226:dbl)
        n107 = Negate(x=w218) -> (-x=w241:dbl)
        n108 = Compound Arithmetic op=ADD(w226, w225, w224, w223) -> (w246:dbl)
        n109 = Multiply(x=0.26666, y=w241) -> (x*y=w239:dbl)
        n110 = Divide(x=w246, y=4.0) -> (x/y=w244:dbl)
        n111 = call-poly <vilib>:"PID.vi"("output range"=cluster{"output high":dbl, "output low":dbl} {"output high"=1.0, "output low"=-1.0}, "PID gains"="Drive to Angle(Distance)", "process variable"=w229, "setpoint"=0.0) -> ("output"=w207:dbl)  [unwired: 6 in, 1 out]
        n112 = Multiply(x=4.0 ("y"), y=3.141592653589793) -> (x*y=w234:dbl)
        n113 = disable-structure shown="Enabled" {
          disable-tunnel: w244 -> [w274 w280]
          disable-tunnel: w234 -> [w272 w279]
          disable-tunnel: [w269 w275] -> w219
          frame Disabled {
            n114 = Divide(x=w274, y=w272) -> (x/y=w273:dbl)
            n115 = Absolute Value(x=w273) -> (abs(x)=w270:dbl)
            n116 = Multiply(x=w270, y=1.34) -> (x*y=w269:dbl)
          }
          frame Enabled {
            n117 = Multiply(x=w280, y=w279) -> (x*y=w277:dbl)
            n118 = Divide(x=w277, y=6.7) -> (x/y=w278:dbl)
            n119 = Absolute Value(x=w278) -> (abs(x)=w275:dbl)
          }
        }
        n120 = Absolute Value(x=w239) -> (abs(x)=w222:dbl)
        n121 = Absolute Value(x=w229) -> (abs(x)=w231:dbl)
        n122 = Subtract(x=w219, y=w222) -> (x-y=w220:dbl)
        n123 = Absolute Value(x=w220) -> (abs(x)=w201:dbl)
        n124 = Less?(x=w231, y=2.0) -> (x < y?=w230:bool)
        n125 = Subtract(x=w221, y=w201) -> (x-y=w191:dbl)
        n126 = call-poly <vilib>:"PID.vi"("output range"=cluster{"output high":dbl, "output low":dbl} {"output high"=1.0, "output low"=-1.0}, "PID gains"="Drive to Angle(Distance)", "process variable"=w191, "setpoint"=0.0) -> ("output"=w204:dbl)  [unwired: 6 in, 1 out]
        n127 = Absolute Value(x=w191) -> (abs(x)=w190:dbl)
        n128 = Less?(x=w190, y=7.0) -> (x < y?=w210:bool)
        n129 = Multiply(x=w208, y=w204) -> (x*y=w209:dbl)
        n130 = Compound Arithmetic op=AND(w210, w230) -> (w242:bool)
        n131 = global write "Robot Global Data.vi" "LED STATE"(enum16{"NORMAL", "RAINBOW"}."NORMAL" ("LED STATE")) -> ()
        n132 = Multiply(x=w205, y=w204) -> (x*y=w206:dbl)
        n133 = case shown="True" w242 {
          tunnel: [FALSE ("ignore previous (F)") TRUE ("ignore previous (F)")] -> w203
          frame False {
          }
          frame True {
          }
        }
        n134 = call "SwerveDrive2.0.vi"("Right Trigger"=w266, "RCW"=w207, "STR"=w206, "FWD"=w209, "Gyro"=w216) -> ()  [unwired: 7 in]
      }
      frame "Stop" {
        n135 = call <vilib>:"WPI_MotorControlRefNum Registry Get.vi"("refnum name"="W3 Power") -> ("error out"=w305:errorcluster, "MotorControlDevRef"=w304:T20)  [unwired: 9 in]
        n136 = call <vilib>:"WPI_MotorControlRefNum Registry Get.vi"("refnum name"="W2 Power") -> ("MotorControlDevRef"=w306:T20)  [unwired: 9 in, 1 out]
        n137 = call <vilib>:"WPI_MotorControlRefNum Registry Get.vi"("refnum name"="W4 Power") -> ("error out"=w303:errorcluster, "MotorControlDevRef"=w302:T20)  [unwired: 9 in]
        n138 = call <vilib>:"WPI_MotorControlRefNum Registry Get.vi"("refnum name"="W1 Power") -> ("error out"=w310:errorcluster, "MotorControlDevRef"=w309:T20)  [unwired: 9 in]
        n139 = call <vilib>:"WPI_MotorControlRefNum Registry Get.vi"("refnum name"="W3 Rotation") -> ("error out"=w290:errorcluster, "MotorControlDevRef"=w289:T20)  [unwired: 9 in]
        n140 = call <vilib>:"WPI_MotorControlRefNum Registry Get.vi"("refnum name"="W2 Rotation") -> ("MotorControlDevRef"=w291:T20)  [unwired: 9 in, 1 out]
        n141 = call <vilib>:"WPI_MotorControlRefNum Registry Get.vi"("refnum name"="W4 Rotation") -> ("error out"=w288:errorcluster, "MotorControlDevRef"=w287:T20)  [unwired: 9 in]
        n142 = call <vilib>:"WPI_MotorControlRefNum Registry Get.vi"("refnum name"="W1 Rotation") -> ("error out"=w295:errorcluster, "MotorControlDevRef"=w294:T20)  [unwired: 9 in]
        n143 = call <vilib>:"WPI_MotorControlSetOutput.vi"("error in (no error)"=w288, "Output"=0.0, "MotorControlDevRef"=w287) -> ()  [unwired: 6 in, 3 out]
        n144 = call <vilib>:"WPI_MotorControlSetOutput.vi"("error in (no error)"=w290, "Output"=0.0, "MotorControlDevRef"=w289) -> ()  [unwired: 6 in, 3 out]
        n145 = call <vilib>:"WPI_MotorControlSetOutput.vi"("error in (no error)"=w303, "Output"=0.0, "MotorControlDevRef"=w302) -> ()  [unwired: 6 in, 3 out]
        n146 = call <vilib>:"WPI_MotorControlSetOutput.vi"("error in (no error)"=w295, "Output"=0.0, "MotorControlDevRef"=w294) -> ()  [unwired: 6 in, 3 out]
        n147 = call <vilib>:"WPI_MotorControlSetOutput.vi"("Output"=0.0, "MotorControlDevRef"=w291) -> ()  [unwired: 7 in, 3 out]
        n148 = call <vilib>:"WPI_MotorControlSetOutput.vi"("error in (no error)"=w305, "Output"=0.0, "MotorControlDevRef"=w304) -> ()  [unwired: 6 in, 3 out]
        n149 = call <vilib>:"WPI_MotorControlSetOutput.vi"("error in (no error)"=w310, "Output"=0.0, "MotorControlDevRef"=w309) -> ()  [unwired: 6 in, 3 out]
        n150 = call <vilib>:"WPI_MotorControlSetOutput.vi"("Output"=0.0, "MotorControlDevRef"=w306) -> ()  [unwired: 7 in, 3 out]
      }
      frame "Balance" {
        n151 = call <vilib>:"ADIS16470 RefNum Registry Get.vi"("refnum name"="Gyro") -> ("error out"=w332:errorcluster, "ADIS16470DevRef out"=w331:T9)  [unwired: 9 in]
        n152 = call <vilib>:"ADIS16470 Read.vi"("error in (no error)"=w332, "ADIS16470DevRef"=w331) -> ("ADIS16470 Value"=w330:T19)  [unwired: 6 in, 3 out]
        n153 = Unbundle By Name(w330) -> ("ZAngle"=w326:dbl, "XAngle"=w318:dbl)
        n154 = call-poly <vilib>:"PID.vi"("output range"=cluster{"output high":dbl, "output low":dbl} {"output high"=0.5, "output low"=-0.5}, "PID gains"="Balance", "process variable"=w318, "setpoint"=0.0) -> ("output"=w317:dbl)  [unwired: 6 in, 1 out]
        n155 = Negate(x=w317) -> (-x=w316:dbl)
        n156 = call "SwerveDrive2.0.vi"("Right Trigger"=0.0, "RCW"=0.0, "STR"=0.0, "FWD"=w316, "Gyro"=w326) -> ()  [unwired: 7 in]
        n157 = Absolute Value(x=w318) -> (abs(x)=w322:dbl)
        n158 = Less?(x=w322, y=1.0) -> (x < y?=w315:bool)
        n159 = case shown="False" w315 {
          frame False {
            n160 = global write "Robot Global Data.vi" "LED STATE"(enum16{"NORMAL", "RAINBOW"}."NORMAL" ("LED STATE")) -> ()
          }
          frame True {
            n161 = global write "Robot Global Data.vi" "LED STATE"(enum16{"NORMAL", "RAINBOW"}."RAINBOW" ("LED STATE")) -> ()
          }
        }
      }
      frame "Look At Cone" {
        n162 = flat-sequence {
          tunnel: [w342] -> w335
          frame #0 {
            n163 = global write "Robot Global Data.vi" "target"(T8."Cone" ("target")) -> ()
          }
          frame #1 {
            n164 = call <vilib>:"ADIS16470 RefNum Registry Get.vi"("refnum name"="Gyro") -> ("error out"=w345:errorcluster, "ADIS16470DevRef out"=w346:T9)  [unwired: 9 in]
            n165 = global read "Robot Global Data.vi" "VisionAngle"() -> (w338:dbl)
            n166 = call <vilib>:"ADIS16470 Read.vi"("error in (no error)"=w345, "ADIS16470DevRef"=w346) -> ("ADIS16470 Value"=w347:T19)  [unwired: 6 in, 3 out]
            n167 = Unbundle By Name(w347) -> ("ZAngle"=w348:dbl)
            n168 = Absolute Value(x=w338) -> (abs(x)=w339:dbl)
            n169 = Greater?(x=w339, y=20.0) -> (0:w340:bool)
            n170 = case shown="True" w340 {
              tunnel: w348 -> [_ w356]
              tunnel: w338 -> [_ w350]
              frame False {
              }
              frame True {
                (unwired) 160.0 ("x")
                n171 = call-poly <vilib>:"PID.vi"("output range"=cluster{"output high":dbl, "output low":dbl} {"output high"=0.1, "output low"=-0.1}, "PID gains"="Look At Cone", "process variable"=w350, "setpoint"=0.0) -> ("output"=w357:dbl)  [unwired: 6 in, 1 out]
                n172 = Negate(x=w357) -> (-x=w359:dbl)
                n173 = call "SwerveDrive2.0.vi"("Right Trigger"=0.0, "RCW"=w359, "STR"=0.0, "FWD"=0.0, "Gyro"=w356) -> ()  [unwired: 7 in]
              }
            }
            n174 = Absolute Value(x=w338) -> (abs(x)=w349:dbl)
            n175 = Less?(x=w349, y=20.0) -> (x < y?=w342:bool)
          }
        }
      }
      frame "Look At Cube" {
        n176 = flat-sequence {
          tunnel: [w367] -> w360
          frame #0 {
            n177 = global write "Robot Global Data.vi" "target"(T8."Cube" ("target")) -> ()
          }
          frame #1 {
            n178 = global read "Robot Global Data.vi" "VisionAngle"() -> (w366:dbl)
            n179 = call <vilib>:"ADIS16470 RefNum Registry Get.vi"("refnum name"="Gyro") -> ("error out"=w370:errorcluster, "ADIS16470DevRef out"=w371:T9)  [unwired: 9 in]
            n180 = call <vilib>:"ADIS16470 Read.vi"("error in (no error)"=w370, "ADIS16470DevRef"=w371) -> ("ADIS16470 Value"=w372:T19)  [unwired: 6 in, 3 out]
            n181 = Absolute Value(x=w366) -> (abs(x)=w365:dbl)
            n182 = Unbundle By Name(w372) -> ("ZAngle"=w373:dbl)
            n183 = Greater?(x=w365, y=15.0) -> (0:w363:bool)
            n184 = case shown="True" w363 {
              tunnel: w366 -> [_ w385]
              tunnel: w373 -> [_ w381]
              frame False {
                n185 = call "Swerve.vi"("SubSystem Data"=T2 {"Operation"=enum."Stop", "Gyro"=0.0, "FWD"=0.0, "STR"=0.0, "X rotate"=0.0, "Y rotate"=0.0, "Time"=0.0, "Distance"=0.0, "Right Trigger"=0.0, "Angle"=0.0, "Start Angle"=0.0, "Tag ID"=0.0, "Start Positions"=[]}) -> ()  [unwired: 10 in, 1 out]
              }
              frame True {
                n186 = call-poly <vilib>:"PID.vi"("output range"=cluster{"output high":dbl, "output low":dbl} {"output high"=0.5, "output low"=-0.5}, "PID gains"="Look At Cube", "process variable"=w385, "setpoint"=0.0) -> ("output"=w382:dbl)  [unwired: 6 in, 1 out]
                n187 = Negate(x=w382) -> (-x=w384:dbl)
                n188 = call "SwerveDrive2.0.vi"("Right Trigger"=0.0, "RCW"=w384, "STR"=0.0, "FWD"=0.0, "Gyro"=w381) -> ()  [unwired: 7 in]
              }
            }
            n189 = Absolute Value(x=w366) -> (abs(x)=w374:dbl)
            n190 = Less?(x=w374, y=15.0) -> (x < y?=w367:bool)
          }
        }
      }
      frame "Move To Tag" {
        n191 = flat-sequence {
          tunnel: w389 -> [w391]
          tunnel: [w391] -> w386
          tunnel: [w392] -> w388
          tunnel: w386 -> [w395]
          frame #0 {
            n192 = global write "Robot Global Data.vi" "target"(T8."AprilTag" ("target")) -> ()
          }
          frame #1 {
            n193 = global read "Robot Global Data.vi" "Detected Tags"() -> (w396:T24)
            n194 = for {
              tunnel: w396 -> [w406] mode=indexing
              tunnel: w395 -> [w404]
              tunnel: [w401] -> w394 mode=indexing
              n195 = Unbundle By Name(w406) -> ("Center.X"=w403:dbl, "tag ID"=w405:i32)
              n196 = Equal?(x=w405, y=w404) -> (x = y?=w402:bool)
              n197 = case shown="True" w402 {
                tunnel: w403 -> [_ w420]
                tunnel: [0.0 w408] -> w401
                frame False {
                }
                frame True {
                  n198 = Subtract(x=w420, y=160.0 ("x")) -> (x-y=w408:dbl)
                  n199 = call-poly <vilib>:"PID.vi"("output range"=cluster{"output high":dbl, "output low":dbl} {"output high"=0.1, "output low"=-0.1}, "PID gains"="AprilTag", "process variable"=w408, "setpoint"=0.0) -> ("output"=w422:dbl)  [unwired: 6 in, 1 out]
                  n200 = call <vilib>:"ADIS16470 RefNum Registry Get.vi"("refnum name"="Gyro") -> ("error out"=w415:errorcluster, "ADIS16470DevRef out"=w416:T9)  [unwired: 9 in]
                  n201 = call <vilib>:"ADIS16470 Read.vi"("error in (no error)"=w415, "ADIS16470DevRef"=w416) -> ("ADIS16470 Value"=w417:T19)  [unwired: 6 in, 3 out]
                  n202 = Unbundle By Name(w417) -> ("ZAngle"=w413:dbl)
                  n203 = call "SwerveDrive2.0.vi"("Right Trigger"=0.0, "RCW"=0.0, "STR"=w422, "FWD"=0.0, "Gyro"=w413) -> ()  [unwired: 7 in]
                }
              }
            }
            n204 = for {
              tunnel: [w400] -> w393 mode=indexing
              tunnel: w394 -> [w399] mode=indexing
              n205 = Absolute Value(x=w399) -> (abs(x)=w398:dbl)
              n206 = Less?(x=w398, y=10.0) -> (x < y?=w400:bool)
            }
            n207 = And Array Elements(Boolean array=w393) -> (logical AND=w392:bool)
          }
        }
      }
      frame "Move To Tape" {
        n208 = flat-sequence {
          tunnel: [w426] -> w424
          frame #0 {
            n209 = global write "Robot Global Data.vi" "target"(T8."Reflective Tape" ("target")) -> ()
          }
          frame #1 {
            n210 = global read "Robot Global Data.vi" "VisionAngle"() -> (w429:dbl)
            n211 = call <vilib>:"ADIS16470 RefNum Registry Get.vi"("refnum name"="Gyro") -> ("error out"=w436:errorcluster, "ADIS16470DevRef out"=w437:T9)  [unwired: 9 in]
            n212 = call <vilib>:"ADIS16470 Read.vi"("error in (no error)"=w436, "ADIS16470DevRef"=w437) -> ("ADIS16470 Value"=w438:T19)  [unwired: 6 in, 3 out]
            n213 = Unbundle By Name(w438) -> ("ZAngle"=w434:dbl)
            n214 = call-poly <vilib>:"PID.vi"("output range"=cluster{"output high":dbl, "output low":dbl} {"output high"=0.1, "output low"=-0.1}, "PID gains"="Tape", "process variable"=w429, "setpoint"=0.0) -> ("output"=w441:dbl)  [unwired: 6 in, 1 out]
            n215 = Absolute Value(x=w429) -> (abs(x)=w428:dbl)
            n216 = Less?(x=w428, y=10.0) -> (x < y?=w426:bool)
            n217 = call "SwerveDrive2.0.vi"("Right Trigger"=0.0, "RCW"=0.0, "STR"=w441, "FWD"=0.0, "Gyro"=w434) -> ()  [unwired: 7 in]
          }
        }
      }
    }
    n218 = call "Swerve Check for New Command.vi"("Current Command"=w18, "Wait time (ms)"=w23, "Finished?"=w6) -> ("Completion"=w19:T4, "Subsystem Name"=w20:string, "Current Command"=w21:T2, "Initial Trace String"=w22:string, "NextCommand"=w24:T7)  [unwired: 4 in]
    n219 = case shown="\"Successful\", \"Aborted\"" w19 {
      selector: w19 -> [_ w449]
      tunnel: w22 -> [_ w445]
      tunnel: w21 -> [_ w446]
      tunnel: w20 -> [_ w442]
      frame "Incomplete", Default {
        # "Continuing current command"
      }
      frame "Successful", "Aborted" {
        # "Report and setup for next command"
        n220 = Unbundle By Name(w446) -> ("Gyro"=w448:dbl, "Y rotate"=w443:dbl)
        n221 = Format Into String(format string="S %.1f, D %f", initial string=w445, w448, w443) -> (resulting string=w444:string)  [unwired: 1 in, 1 out]
        "Current\nCmd" <- w444
        n222 = call <vilib>:"Trace Results.vi"("Status of previous command"=w449, "Description"=w444, "Subsystem"=w442) -> ()  [unwired: 9 in]
      }
    }
    n223 = disable-structure shown="Disabled" {
      frame Disabled {
        # "Publish"
        n224 = call-poly <vilib>:"NT Write Value.vi"() -> ()  [unwired: 11 in, 1 out]
      }
      frame Enabled {
      }
    }
  }
  n225 = while {
    tunnel: w1 -> [w456]
    stop <- FALSE stop-if-true
    n226 = call "Swerve Controller Interactive Check.vi"("Interactive Command in"="Interactive Values", "Default Command"=w456, "Buttons"="Buttons") -> ("Interactive Command out"=w453:T2, "Trace String"=w454:string, "Schedule"=w455:bool)  [unwired: 6 in]
    n227 = case shown="True" w455 {
      tunnel: [w467 w472] -> w452
      tunnel: w453 -> [_ w470]
      tunnel: [w463 w468] -> w451
      tunnel: w454 -> [_ w471]
      frame False {
        n228 = Tick Count (ms)() -> (millisecond timer value=w462:u32)
        n229 = call "Read Swerve Operation.vi"() -> ("Command Info"=w460:T5, "SubSystem Data"=w461:T2)  [unwired: 9 in, 1 out]
        n230 = Unbundle(w461) -> ("Operation"=w466:T3, "Gyro"=w464:dbl)  [unwired: 11 out]
        n231 = Unbundle(w460) -> ("Status"=w467:T4)  [unwired: 2 out]
        n232 = Subtract(x=w462, y=w466) -> (x-y=w465:u32)
        n233 = Bundle(w465, "Gyro"=w464) -> (w463:cluster{u32, "Gyro":dbl})  [unwired: 1 in]
      }
      frame True {
        n234 = call "Swerve Command Helper.vi"("Description"=w471, "SubSystem Data"=w470) -> ("Command Info Out"=w469:T5, "Command Timing"=w468:cluster{"Start Time (ms)":u32, "Iterations":i32})  [unwired: 7 in, 1 out]
        n235 = Unbundle(w469) -> ("Status"=w472:T4)  [unwired: 2 out]
      }
    }
    "Status" <- w452
    "Command Timing" <- w451
    n236 = Wait (ms)(milliseconds to wait=u32 20) -> ()  [unwired: 1 out]
  }
